vi "LaserCal-Options Dialog.vi"(0 "Cluster In":T2, 2 "Parent VI":refnum<vi>) -> (4 "Cluster out":T2, 8 "Canceled?":bool)   [LabVIEW 2015]
uses:
  Typedefs/LaserCal-Options.ctl
  Utility VIs/Buttons/KCheckmarkBoolean 2.ctl
panel:
  in  "mA/V":dbl caption="Current source sensitivity (mA/V)"
  in  "save current":T1 caption="Save calibration in current units"
  in  "current":T1 caption="Express input in current units"
  in  "Cancel":bool
  in  "OK":bool
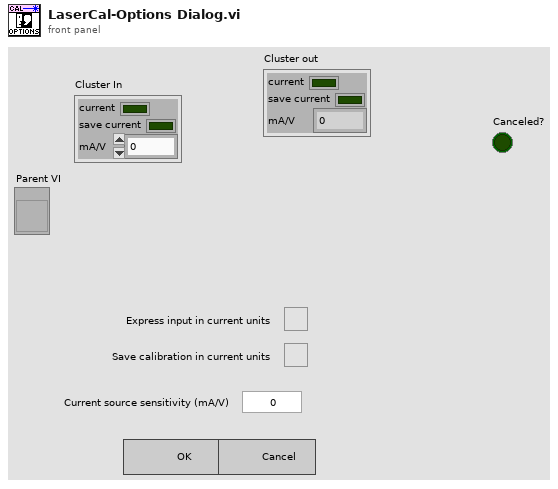
[diagram p1: front panel]
types:
  T1 = typedef "KCheckmarkBoolean 2.ctl" = bool
  T2 = typedef "LaserCal-Options.ctl" = cluster{"current":bool, "save current":bool, "mA/V":dbl}
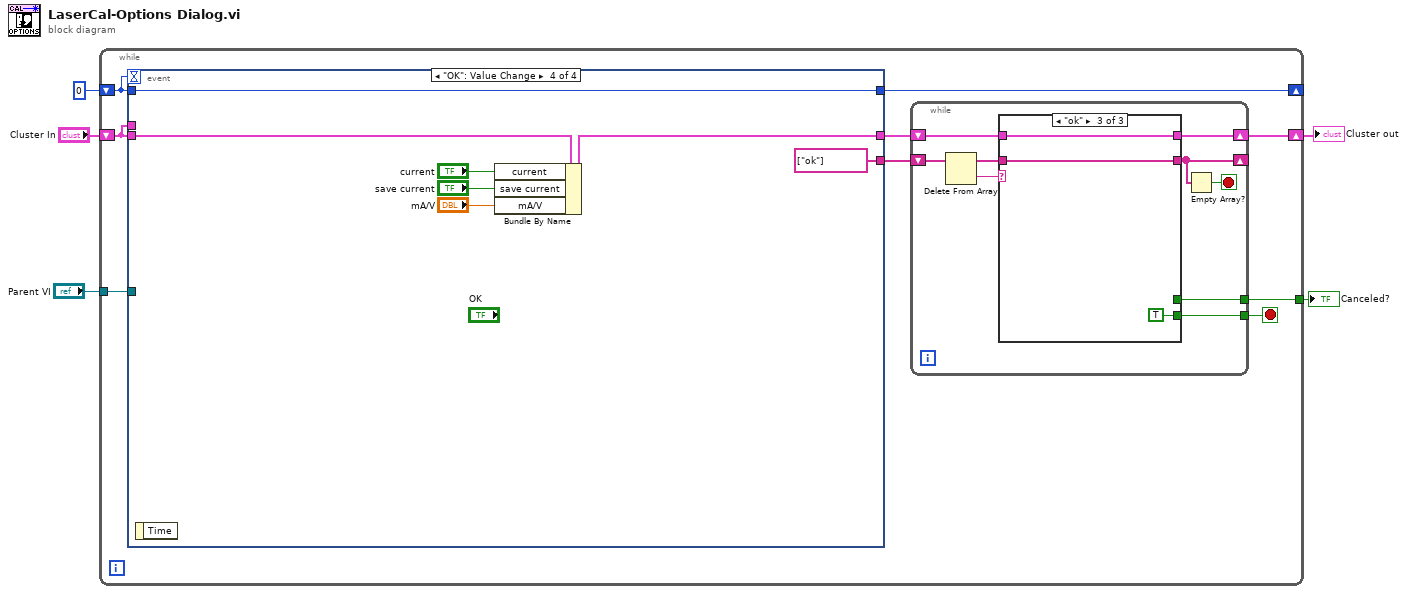
[diagram p0: block diagram]
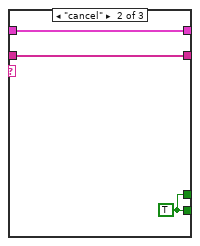
[diagram p3: hidden frame]
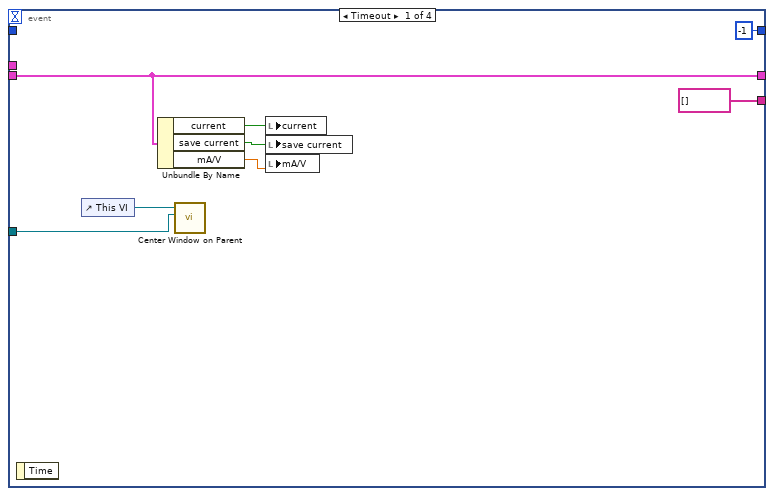
[diagram p4: hidden frame]
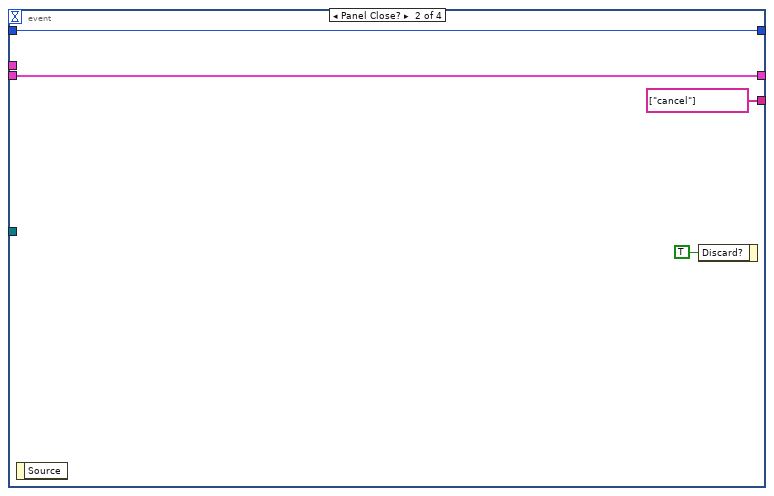
[diagram p5: hidden frame]
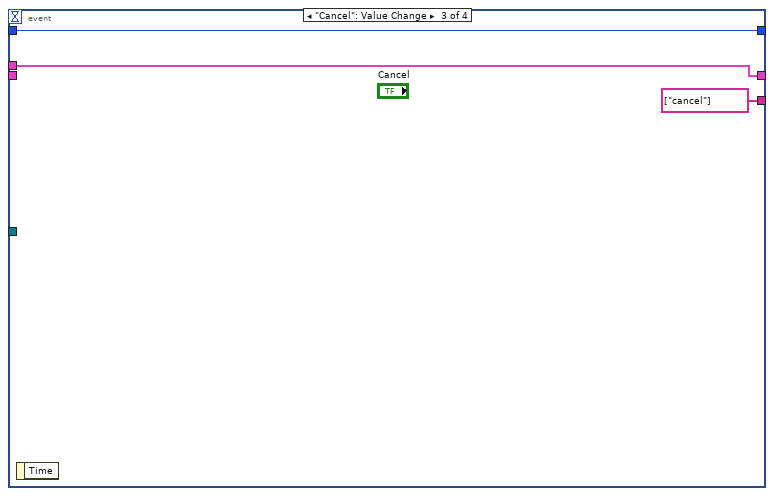
[diagram p6: hidden frame]
diagram:
  n1 = while {
    shift-right: [w14] -> _
    shift-left: 0 -> [w12]
    tunnel: [w7] -> w2
    shift-right: [w8] -> w3
    shift-left: "Cluster In" -> [w13]
    tunnel: "Parent VI" -> [w6]
    stop <- w9 stop-if-true
    n2 = event shown="[3] \"OK\": Value Change" {
      selector: _ -> [_ _ _ _]
      dyn-events: _ -> [_ _ _ _]
      timeout: w12 -> [_ _ _ _]
      tunnel: [-1 w43 w45 w52] -> w14
      tunnel: w13 -> [w35 w42 _ w53]
      tunnel: [w35 w42 w46 w50] -> w11
      tunnel: w13 -> [_ _ w46 _]
      tunnel: w12 -> [_ w43 w45 w52]
      tunnel: [string[] [] string[] ["cancel"] string[] ["cancel"] string[] ["ok"]] -> w10
      tunnel: w6 -> [w36 _ _ _]
      event Timeout {
        n3 = event-data() -> ()  [unwired: 1 in, 1 out]
        n4 = control-ref of="This VI"() -> (w37:refnum<vi>)
        n5 = Unbundle By Name(w35) -> ("current"=w34:bool, "save current"=w33:bool, "mA/V"=w32:dbl)
        n6 = call "Center Window on Parent.vi"("Parent VI"=w36, "VI in"=w37) -> ()  [unwired: 8 in, 2 out]
        n7 = local write "current"(w34) -> ()
        n8 = local write "save current"(w33) -> ()
        n9 = local write "mA/V"(w32) -> ()
      }
      event Panel Close? {
        n10 = event-data() -> ()  [unwired: 1 in, 1 out]
        n11 = event-data("Discard?"=TRUE) -> ()  [unwired: 1 in, 1 out]
      }
      event "Cancel": Value Change {
        n12 = event-data() -> ()  [unwired: 1 in, 1 out]
      }
      event "OK": Value Change {
        n13 = event-data() -> ()  [unwired: 1 in, 1 out]
        n14 = Bundle By Name(cluster=w53, "current"="current", "save current"="save current", "mA/V"="mA/V") -> (w50:T2)
      }
    }
    n15 = while {
      shift-right: [w20] -> _
      shift-left: w10 -> [w23]
      shift-right: [w17] -> w8
      shift-left: w11 -> [w18]
      tunnel: [w16] -> w9
      tunnel: [w15] -> w7
      stop <- w19 stop-if-true
      n16 = Delete From Array(array=w23) -> (deleted portion=w21:string, array with subset deleted=w22:string[])  [unwired: 2 in]
      n17 = case shown="\"ok\"" w21 {
        tunnel: w22 -> [w25 w28 w31]
        tunnel: [w25 w28 w31] -> w20
        tunnel: w18 -> [w24 w27 w30]
        tunnel: [w24 w27 w30] -> w17
        tunnel: [_ w26 TRUE] -> w16
        tunnel: [_ w26 _] -> w15
        frame "", Default {
        }
        frame "cancel" {
          w26 = TRUE
        }
        frame "ok" {
        }
      }
      n18 = Empty Array?(array=w20) -> (empty?=w19:bool)
    }
  }
  "Cluster out" <- w3
  "Canceled?" <- w2
